vi "test_libssh2_session_last_error.vi"() -> ()   [LabVIEW 2017, in "unit_tests.lvlib"]
uses:
  unit_tests.lvlib
  libssh2/libssh2_init_default.vi
  libssh2/libssh2_session_init_ex.vi
  libssh2/libssh2.lvlib
  <vilib>/PNR/Transparent Assertions/Transparent Assertions/Transparent Assertions.lvlib
panel:
  out "error out":errorcluster
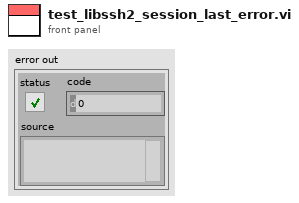
[diagram p1: front panel]
types:
  T1 = typedef "libssh2.lvlib/Session Refnum.ctl" = refnum<k1>
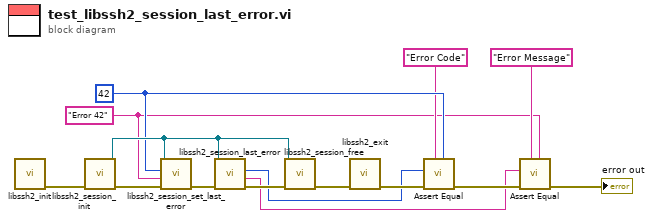
[diagram p0: block diagram]
diagram:
  w1 = "Error 42"
  w7 = 42 ("timeout in ms (0 = indefinite)")
  n1 = call-poly "libssh2_init.vi"() -> ("error out"=w15:errorcluster)  [unwired: 11 in]
  n2 = call "libssh2_session_init.vi"("error in (no error)"=w15) -> ("error out"=w8:errorcluster, "session"=w10:T1)  [unwired: 9 in]
  n3 = call "libssh2_session_set_last_error.vi"("error in (no error)"=w8, "error message"=w1, "error code"=w7, "session"=w10) -> ("error out"=w13:errorcluster)  [unwired: 7 in]
  n4 = call "libssh2_session_last_error.vi"("error in (no error)"=w13, "session"=w10) -> ("error out"=w11:errorcluster, "error message"=w2:string, "error code"=w9:i32)  [unwired: 7 in]
  n5 = call "libssh2_session_free.vi"("error in (no error)"=w11, "session"=w10) -> ("error out"=w14:errorcluster)  [unwired: 9 in]
  n6 = call "libssh2_exit.vi"("error in (no error)"=w14) -> ("error out"=w12:errorcluster)  [unwired: 10 in]
  n7 = call <vilib>:"Assert Equal.vi"("Expected"=w7, "Message (\"\")"="Error Code" ("Label"), "error in (no error)"=w12, "Actual"=w9) -> ("error out"=w6:errorcluster)  [unwired: 7 in]
  n8 = call <vilib>:"Assert Equal.vi"("Expected"=w1, "Message (\"\")"="Error Message" ("Label"), "error in (no error)"=w6, "Actual"=w2) -> ("error out"=→"error out":errorcluster)  [unwired: 7 in]
